vi "Message splitter.vi"(5 "Message in":string) -> (0 "Byte 4":string, 1 "Byte 3":string, 2 "Byte 2":string, 3 "Byte 1":string, 8 "Byte 8":string, 9 "Byte 7":string, 10 "Byte 6":string, 11 "Byte 5":string)   [LabVIEW 2014]
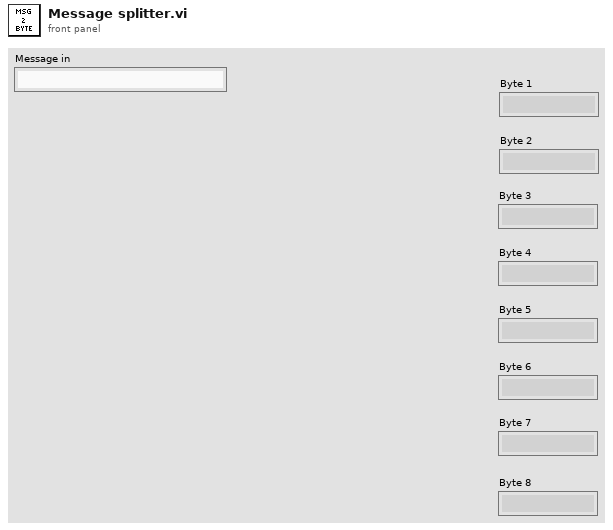
[diagram p1: front panel]
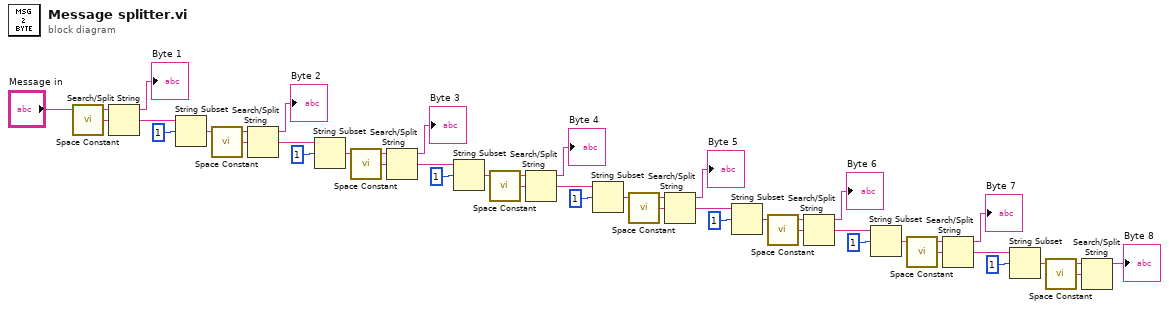
[diagram p0: block diagram]
diagram:
  n1 = call <vilib>:"Space Constant.vi"() -> ("String"=w1:string)
  n2 = Search/Split String(string="Message in", search string/char (-)=w1) -> (substring before match=→"Byte 1":string, match + rest of string=w2:string)  [unwired: 1 in, 1 out]
  n3 = String Subset(string=w2, offset (0)=1) -> (substring=w23:string)  [unwired: 1 in]
  n4 = call <vilib>:"Space Constant.vi"() -> ("String"=w4:string)
  n5 = Search/Split String(string=w23, search string/char (-)=w4) -> (substring before match=→"Byte 2":string, match + rest of string=w5:string)  [unwired: 1 in, 1 out]
  n6 = String Subset(string=w5, offset (0)=1) -> (substring=w24:string)  [unwired: 1 in]
  n7 = call <vilib>:"Space Constant.vi"() -> ("String"=w7:string)
  n8 = Search/Split String(string=w24, search string/char (-)=w7) -> (substring before match=→"Byte 3":string, match + rest of string=w8:string)  [unwired: 1 in, 1 out]
  n9 = String Subset(string=w8, offset (0)=1) -> (substring=w25:string)  [unwired: 1 in]
  n10 = call <vilib>:"Space Constant.vi"() -> ("String"=w10:string)
  n11 = Search/Split String(string=w25, search string/char (-)=w10) -> (substring before match=→"Byte 4":string, match + rest of string=w11:string)  [unwired: 1 in, 1 out]
  n12 = String Subset(string=w11, offset (0)=1) -> (substring=w26:string)  [unwired: 1 in]
  n13 = call <vilib>:"Space Constant.vi"() -> ("String"=w13:string)
  n14 = Search/Split String(string=w26, search string/char (-)=w13) -> (substring before match=→"Byte 5":string, match + rest of string=w14:string)  [unwired: 1 in, 1 out]
  n15 = String Subset(string=w14, offset (0)=1) -> (substring=w27:string)  [unwired: 1 in]
  n16 = call <vilib>:"Space Constant.vi"() -> ("String"=w16:string)
  n17 = Search/Split String(string=w27, search string/char (-)=w16) -> (substring before match=→"Byte 6":string, match + rest of string=w17:string)  [unwired: 1 in, 1 out]
  n18 = String Subset(string=w17, offset (0)=1) -> (substring=w28:string)  [unwired: 1 in]
  n19 = call <vilib>:"Space Constant.vi"() -> ("String"=w19:string)
  n20 = Search/Split String(string=w28, search string/char (-)=w19) -> (substring before match=→"Byte 7":string, match + rest of string=w20:string)  [unwired: 1 in, 1 out]
  n21 = String Subset(string=w20, offset (0)=1) -> (substring=w35:string)  [unwired: 1 in]
  n22 = call <vilib>:"Space Constant.vi"() -> ("String"=w36:string)
  n23 = Search/Split String(string=w35, search string/char (-)=w36) -> (substring before match=→"Byte 8":string)  [unwired: 1 in, 2 out]
